vi "散斑图像作用模块.vi"(9 "散斑矩阵":dbl[][](array[numeric]), 10 "散斑行数":i32, 11 "图像矩阵":dbl[](array[numeric])) -> (3 "纠缠后输出":dbl[](array[numeric]))   [LabVIEW 2018]
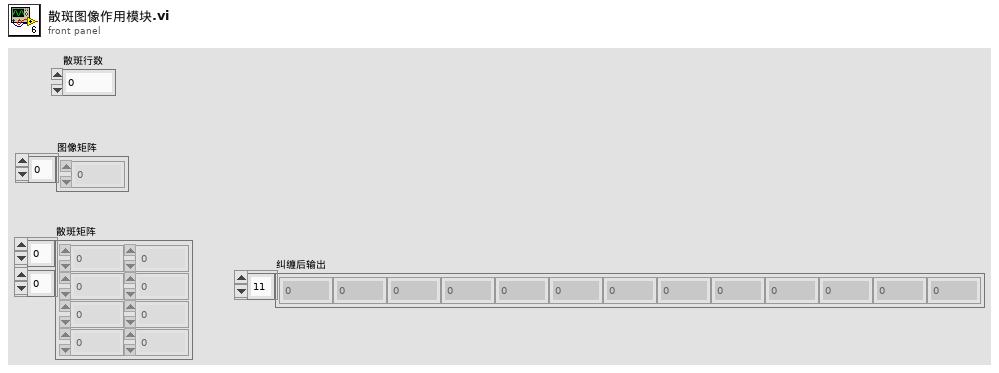
[diagram p1: front panel]
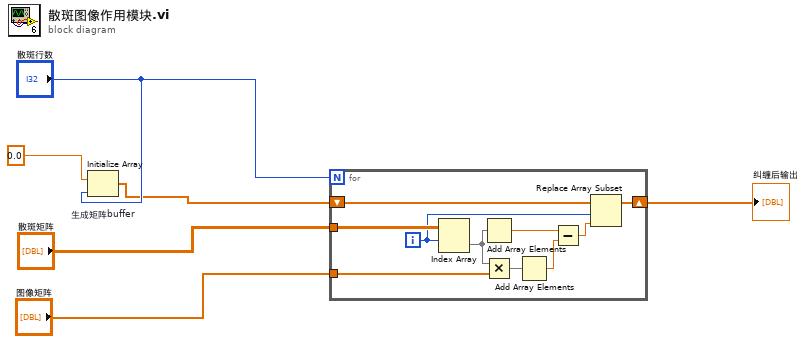
[diagram p0: block diagram]
diagram:
  n1 = Initialize Array "生成矩阵buffer"(0.0, "散斑行数") -> (w1:dbl[])
  n2 = for {
    N: "散斑行数" -> [_]
    tunnel: "图像矩阵" -> [w15]
    tunnel: "散斑矩阵" -> [w16]
    shift-right: [w7] -> w6
    shift-left: w1 -> [w9]
    i -> [w8]
    n3 = Index Array(array=w16, index (row)=w8) -> (element=w13:dbl[])  [unwired: 1 in]
    n4 = Add Array Elements(numeric array=w13) -> (sum=w12:dbl)
    n5 = Multiply(x=w13, y=w15) -> (x*y=w14:dbl[])
    n6 = Add Array Elements(numeric array=w14) -> (sum=w11:dbl)
    n7 = Subtract(x=w12, y=w11) -> (x-y=w10:dbl)
    n8 = Replace Array Subset(array=w9, new element=w10, index=w8) -> (w7:dbl[])
  }
  "纠缠后输出" <- w6
